vi "ReadWriteSettingsFile4.vi"(5 "file path":path, 6 "Read/write":enum16{"Query & Read", "Assign & Read", "Write"}(ring), 9 "Settings In":T1={"Pre-I hold"={"Fixed (s)"=0.5, "Random (s)"=0.5}, "LED I duration"={"Fixed (s)"=0.5, "Random (s)"=0.0}, "All Flash?"=FALSE, "Pre-cue brightness"=0, "Post-I hold"={"Fixed (s)"=0.7, "Random (s)"=0.3}, "Post-I \nbounce-off"={"Fixed (s)"=0.3, "Random (s)"=0.0}, "Capture timeout"={"Fixed (s)"=1.5, "Random (s)"=0.0}, "Tone duration"={"Fixed (s)"=0.5, "Random (s)"=0.0}, "LED C duration"={"Fixed (s)"=0.5, "Random (s)"=0.0}, "Cue brightness"=0, "Hold duration"={"Fixed (s)"=0.3, "Random (s)"=0.0}, "Allowed\nbounce-off"={"Fixed (s)"=0.2, "Random (s)"=0.0}, "Post-capture brightness"=0, "Reward duration"={"Fixed (s)"=0.7, "Random (s)"=0.0}, "Intertrial interval"={"Fixed (s)"=0.5, "Random (s)"=0.0}, "Persistent Mode?"=FALSE, "Error bong?"=TRUE, "Critter"=0, "Blocks"=[], "Target set"=[], "Rand/Seq?"=TRUE, "Trial type"=0, "Sines?"=FALSE, "Bumps"=FALSE, "Sine parameters"={"Frequency"=0.25, "Degrees\npk-pk"=6.0, "Cycles"=10000}, "Bump timing"={"Fix"=2.0, "Rnd"=8.0}, "Bump Parameters"={"Distance (deg)"=2.0, "Travel time (ms)"=500.0}, "DBS On?"=FALSE, "Home reward?"=FALSE, "Home+target OK?"=FALSE} {"Bump Parameters"."Travel time (ms)" min=0.1 max=10000.0; "Bump Parameters"."Distance (deg)" min=0.1; "Bump timing"."Rnd" format="%.4f"; "Bump timing"."Fix" format="%_4g"; "Sine parameters"."Degrees\npk-pk" min=0.1 max=120.0; "Sine parameters"."Frequency" min=0.001 format="%#_4g"; "Trial type" items=["Allflash/sensory", "Precue/memory"]; "Target set" items=["1", "2", "3", "4"]; "Critter" items=["Mojo", "Smokey"]; "Post-I \nbounce-off"."Random (s)" format="%.4f"; "Post-I \nbounce-off"."Fixed (s)" format="%_4g"; "Allowed\nbounce-off"."Random (s)" format="%.4f"; "Allowed\nbounce-off"."Fixed (s)" format="%_4g"; "LED C duration"."Random (s)" format="%.4f"; "LED C duration"."Fixed (s)" format="%.4f"; "Capture timeout"."Random (s)" format="%.4f"; "Capture timeout"."Fixed (s)" format="%.4f"; "Post-I hold"."Random (s)" format="%.4f"; "Post-I hold"."Fixed (s)" format="%.4f"; "Hold duration"."Random (s)" format="%.4f"; "Hold duration"."Fixed (s)" format="%_4g"; "Intertrial interval"."Random (s)" format="%.4f"; "Intertrial interval"."Fixed (s)" format="%.4f"; "Reward duration"."Random (s)" format="%.4f"; "Reward duration"."Fixed (s)" format="%.4f"; "LED I duration"."Random (s)" format="%.4f"; "LED I duration"."Fixed (s)" format="%.4f"; "Tone duration"."Random (s)" format="%.4f"; "Tone duration"."Fixed (s)" format="%.4f"; "Pre-I hold"."Random (s)" format="%.4f"; "Pre-I hold"."Fixed (s)" format="%_4g"}) -> (0 "Read Error":errorcluster, 1 "Write error":errorcluster, 3 "Settings Out":T1={"Pre-I hold"={"Fixed (s)"=0.5, "Random (s)"=0.5}, "LED I duration"={"Fixed (s)"=0.5, "Random (s)"=0.0}, "All Flash?"=FALSE, "Pre-cue brightness"=0, "Post-I hold"={"Fixed (s)"=0.7, "Random (s)"=0.3}, "Post-I \nbounce-off"={"Fixed (s)"=0.3, "Random (s)"=0.0}, "Capture timeout"={"Fixed (s)"=1.5, "Random (s)"=0.0}, "Tone duration"={"Fixed (s)"=0.5, "Random (s)"=0.0}, "LED C duration"={"Fixed (s)"=0.5, "Random (s)"=0.0}, "Cue brightness"=0, "Hold duration"={"Fixed (s)"=0.3, "Random (s)"=0.0}, "Allowed\nbounce-off"={"Fixed (s)"=0.2, "Random (s)"=0.0}, "Post-capture brightness"=0, "Reward duration"={"Fixed (s)"=0.7, "Random (s)"=0.0}, "Intertrial interval"={"Fixed (s)"=0.5, "Random (s)"=0.0}, "Persistent Mode?"=FALSE, "Error bong?"=TRUE, "Critter"=0, "Blocks"=[], "Target set"=[], "Rand/Seq?"=TRUE, "Trial type"=0, "Sines?"=FALSE, "Bumps"=FALSE, "Sine parameters"={"Frequency"=0.25, "Degrees\npk-pk"=6.0, "Cycles"=10000}, "Bump timing"={"Fix"=2.0, "Rnd"=8.0}, "Bump Parameters"={"Distance (deg)"=2.0, "Travel time (ms)"=500.0}, "DBS On?"=FALSE, "Home reward?"=FALSE, "Home+target OK?"=FALSE} {"Bump Parameters"."Travel time (ms)" min=0.1 max=10000.0; "Bump Parameters"."Distance (deg)" min=0.1; "Bump timing"."Rnd" format="%.4f"; "Bump timing"."Fix" format="%_4g"; "Sine parameters"."Degrees\npk-pk" min=0.1 max=120.0; "Sine parameters"."Frequency" min=0.001 format="%#_4g"; "Trial type" items=["Allflash/sensory", "Precue/memory"]; "Target set" items=["1", "2", "3", "4"]; "Critter" items=["Mojo", "Smokey"]; "Post-I \nbounce-off"."Random (s)" format="%.4f"; "Post-I \nbounce-off"."Fixed (s)" format="%_4g"; "Allowed\nbounce-off"."Random (s)" format="%.4f"; "Allowed\nbounce-off"."Fixed (s)" format="%_4g"; "LED C duration"."Random (s)" format="%.4f"; "LED C duration"."Fixed (s)" format="%.4f"; "Capture timeout"."Random (s)" format="%.4f"; "Capture timeout"."Fixed (s)" format="%.4f"; "Post-I hold"."Random (s)" format="%.4f"; "Post-I hold"."Fixed (s)" format="%.4f"; "Hold duration"."Random (s)" format="%.4f"; "Hold duration"."Fixed (s)" format="%_4g"; "Intertrial interval"."Random (s)" format="%.4f"; "Intertrial interval"."Fixed (s)" format="%.4f"; "Reward duration"."Random (s)" format="%.4f"; "Reward duration"."Fixed (s)" format="%.4f"; "LED I duration"."Random (s)" format="%.4f"; "LED I duration"."Fixed (s)" format="%.4f"; "Tone duration"."Random (s)" format="%.4f"; "Tone duration"."Fixed (s)" format="%.4f"; "Pre-I hold"."Random (s)" format="%.4f"; "Pre-I hold"."Fixed (s)" format="%_4g"}, 4 "current path":path)   [LabVIEW 2010]
panel:
  # "Pre-\ninstruction\nhold"
  # "Instruction"
  # "Post-\ninstruction\nhold"
  # "Target capture"
  # "Target hold"
  # "Reward"
  # "Intertrial"
  # "+"
  # "Pre-\ninstruction\nhold"
  # "Instruction"
  # "Post-\ninstruction\nhold"
  # "Target capture"
  # "Target hold"
  # "Reward"
  # "Intertrial"
  # "+"
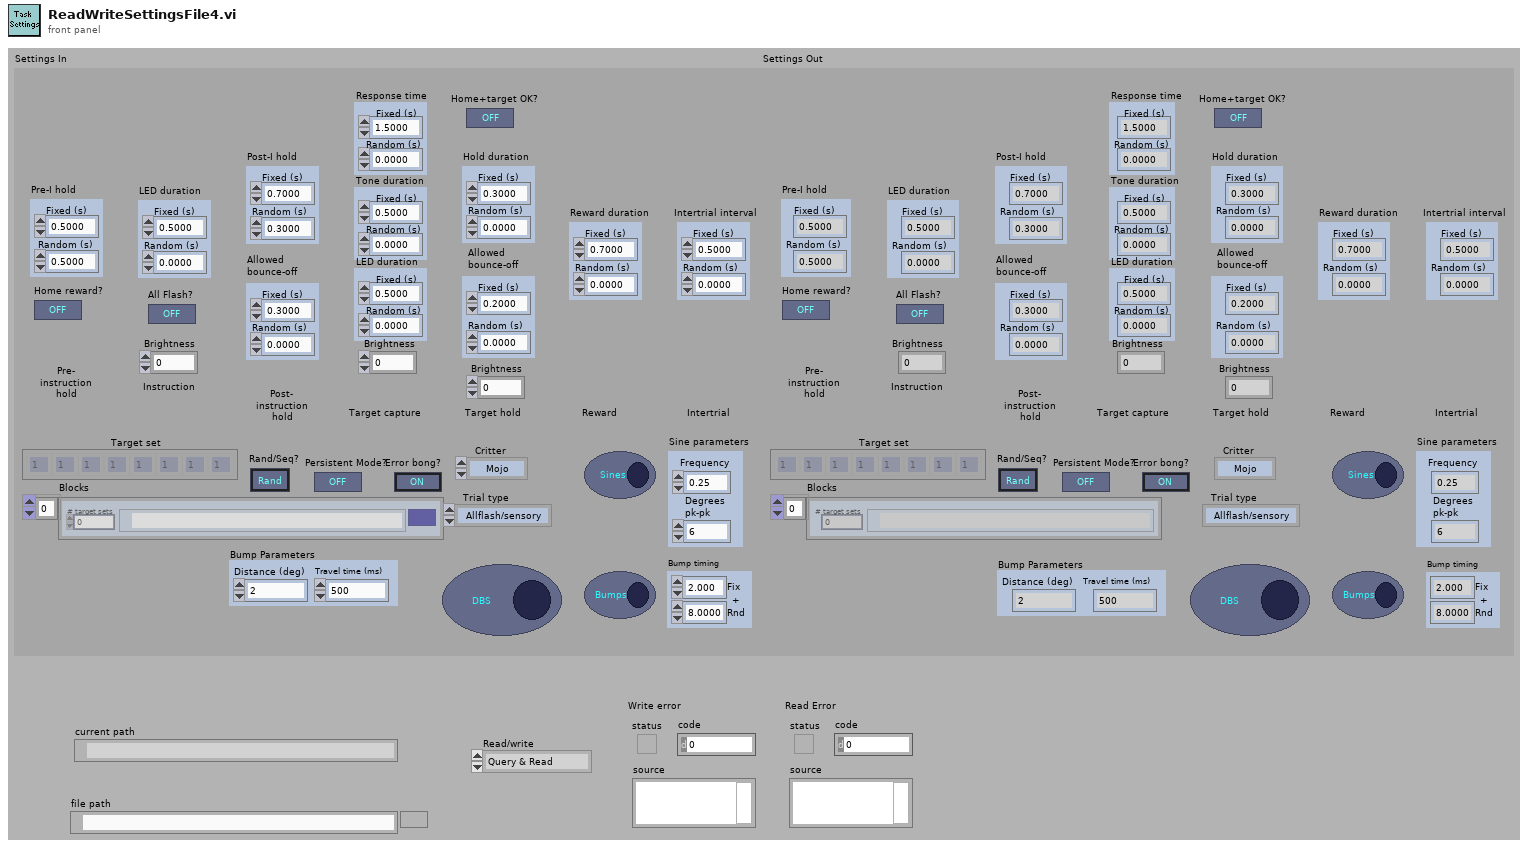
[diagram p1: front panel]
types:
  T1 = cluster{"Pre-I hold":cluster{"Fixed (s)":dbl, "Random (s)":dbl}, "LED I duration":cluster{"Fixed (s)":dbl, "Random (s)":dbl}, "All Flash?":bool, "Pre-cue brightness":i16, "Post-I hold":cluster{"Fixed (s)":dbl, "Random (s)":dbl}, "Post-I \nbounce-off":cluster{"Fixed (s)":dbl, "Random (s)":dbl}, "Capture timeout":cluster{"Fixed (s)":dbl, "Random (s)":dbl}, "Tone duration":cluster{"Fixed (s)":dbl, "Random (s)":dbl}, "LED C duration":cluster{"Fixed (s)":dbl, "Random (s)":dbl}, "Cue brightness":i16, "Hold duration":cluster{"Fixed (s)":dbl, "Random (s)":dbl}, "Allowed\nbounce-off":cluster{"Fixed (s)":dbl, "Random (s)":dbl}, "Post-capture brightness":i16, "Reward duration":cluster{"Fixed (s)":dbl, "Random (s)":dbl}, "Intertrial interval":cluster{"Fixed (s)":dbl, "Random (s)":dbl}, "Persistent Mode?":bool, "Error bong?":bool, "Critter":u16, "Blocks":cluster{"Settings file":path, "# target sets":dbl}[], "Target set":i16[], "Rand/Seq?":bool, "Trial type":u16, "Sines?":bool, "Bumps":bool, "Sine parameters":cluster{"Frequency":dbl, "Degrees\npk-pk":dbl, "Cycles":i16}, "Bump timing":cluster{"Fix":dbl, "Rnd":dbl}, "Bump Parameters":cluster{"Distance (deg)":dbl, "Travel time (ms)":dbl}, "DBS On?":bool, "Home reward?":bool, "Home+target OK?":bool}
  T2 = enum16{"deny read/write", "deny write-only", "deny none"}
  T3 = enum16{"read/write", "read-only", "write-only", "write-only (truncate)"}
  T4 = enum32{"existing file", "new file", "new or existing file", "existing dir", "new dir", "new or existing dir", "existing file (use LLBs)", "new file (use LLBs)", "new or existing file (use LLBs)", "new or existing file or directory (use LLBs)"}
  T5 = enum16{"open", "replace", "create", "open or create", "replace or create", "replace or create with confirmation"}
  T6 = cluster{"Pre-I hold":cluster{"Fixed (s)":dbl, "Random (s)":dbl}, "LED I duration":cluster{"Fixed (s)":dbl, "Random (s)":dbl}, "All Flash?":bool, "Pre-cue brightness":i16, "Post-I hold":cluster{"Fixed (s)":dbl, "Random (s)":dbl}, "Post-I \nbounce-off":cluster{"Fixed (s)":dbl, "Random (s)":dbl}, "Capture timeout":cluster{"Fixed (s)":dbl, "Random (s)":dbl}, "Tone duration":cluster{"Fixed (s)":dbl, "Random (s)":dbl}, "LED C duration":cluster{"Fixed (s)":dbl, "Random (s)":dbl}, "Cue brightness":i16, "Hold duration":cluster{"Fixed (s)":dbl, "Random (s)":dbl}, "Allowed\nbounce-off":cluster{"Fixed (s)":dbl, "Random (s)":dbl}, "Post-capture brightness":i16, "Reward duration":cluster{"Fixed (s)":dbl, "Random (s)":dbl}, "Intertrial interval":cluster{"Fixed (s)":dbl, "Random (s)":dbl}, "Persistent Mode?":bool, "Error bong?":bool, "Critter":u16, "Blocks":cluster{"Settings file":path, "# target sets":dbl}[], "Target set":i16[], "Rand/Seq?":bool, "Trial type":u16, "Sines?":bool, "Bumps":bool, "Sine parameters":cluster{"Frequency":dbl, "Degrees\npk-pk":dbl, "Cycles":i16}, "Bump timing":cluster{"Fix":dbl, "Rnd":dbl}, "Bump Parameters":cluster{"Distance (deg)":dbl, "Travel time (ms)":dbl}, "DBS On?":bool, "Home reward?":bool, "Home+target OK?":bool}[]
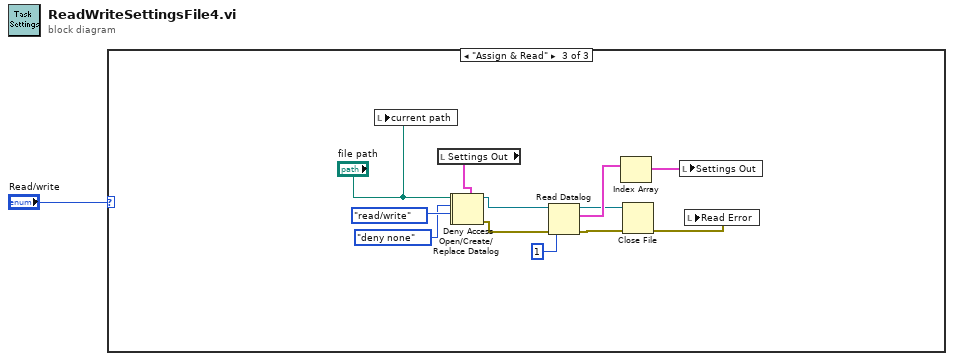
[diagram p0: block diagram]
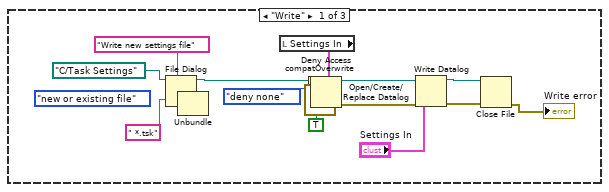
[diagram p2: hidden frame]
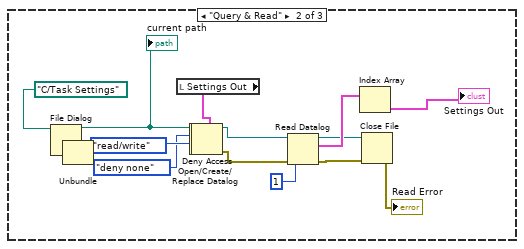
[diagram p3: hidden frame]
diagram:
  n1 = case shown="\"Assign & Read\"" "Read/write" {
    frame "Write" {
      (unwired) T4."new or existing file" ("select mode (2)")
      n2 = File Dialog(6:" *.tsk" ("pattern"), 7:"Write new settings file" ("prompt"), 11:path "C:/Task Settings" ("start path  (Not A Path)")) -> (0:w5:errorcluster, 3:w17:path)  [unwired: 4 in, 2 out]
      n3 = Unbundle(w5) -> ()  [unwired: 3 out]
      n4 = local read "Settings In"() -> (w10:T1)
      n5 = call <vilib>:"compatOverwrite.vi"("overwrite (F)"=TRUE) -> ("overwrite?"=w2:T5)
      n6 = Open/Create/Replace Datalog ("New File")(5:w10, 10:w2, 11:w17) -> (0:w4:errorcluster, 3:w3:refnum<k1>)  [unwired: 3 in, 1 out]
      n7 = Deny Access(4:w4, 6:T2."deny none" ("deny mode (2)"), 7:w3) -> (0:w12:errorcluster, 3:w13:refnum<k1>)
      n8 = Write Datalog(4:w12, 6:"Settings In", 7:w13) -> (0:w8:errorcluster, 3:w9:refnum<k1>)
      n9 = Close File(refnum=w9, error in=w8) -> (error out=→"Write error":errorcluster)  [unwired: 1 out]
    }
    frame "Query & Read" {
      n10 = File Dialog(11:path "C:/Task Settings" ("start path")) -> (0:w21:errorcluster, 3:w22:path)  [unwired: 6 in, 2 out]
      "current path" <- w22
      n11 = Unbundle(w21) -> ()  [unwired: 3 out]
      n12 = local read "Settings Out"() -> (w33:T1)
      n13 = Open/Create/Replace Datalog(5:w33, 9:T3."read/write" ("open mode (0)"), 11:w22) -> (0:w20:errorcluster, 3:w19:refnum<k1>)  [unwired: 3 in, 1 out]
      n14 = Deny Access(4:w20, 6:T2."deny none" ("deny mode (2)"), 7:w19) -> (0:w29:errorcluster, 3:w34:refnum<k1>)
      n15 = Read Datalog(4:w29, 6:1 ("count"), 7:w34) -> (0:w28:errorcluster, 2:w32:T6, 3:w26:refnum<k1>)
      n16 = Index Array(array=w32) -> (element=→"Settings Out":T1)  [unwired: 1 in]
      n17 = Close File(refnum=w26, error in=w28) -> (error out=→"Read Error":errorcluster)  [unwired: 1 out]
    }
    frame "Assign & Read" {
      n18 = local write "current path"("file path") -> ()
      n19 = local read "Settings Out"() -> (w47:T1)
      n20 = Open/Create/Replace Datalog(5:w47, 9:T3."read/write" ("open mode (0)"), 11:"file path") -> (0:w36:errorcluster, 3:w35:refnum<k1>)  [unwired: 3 in, 1 out]
      n21 = Deny Access(4:w36, 6:T2."deny none" ("deny mode (2)"), 7:w35) -> (0:w45:errorcluster, 3:w48:refnum<k1>)
      n22 = Read Datalog(4:w45, 6:1 ("count"), 7:w48) -> (0:w44:errorcluster, 2:w46:T6, 3:w43:refnum<k1>)
      n23 = Index Array(array=w46) -> (element=w39:T1)  [unwired: 1 in]
      n24 = Close File(refnum=w43, error in=w44) -> (error out=w38:errorcluster)  [unwired: 1 out]
      n25 = local write "Settings Out"(w39) -> ()
      n26 = local write "Read Error"(w38) -> ()
    }
  }
